vi "get-wakeup-timestamp.vi"(1 "Tga":dbl format="%#_13g", 2 "Tra":dbl format="%#_13g") -> (0 "wake-up timestamp":timestamp)   [LabVIEW 2021]
panel:
  out "current time":timestamp
  # "pre-determined sleep time\nin seconds"
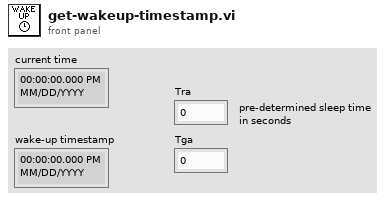
[diagram p1: front panel]
types:
  T1 = typedef "LVDateTimeRec.ctl" = cluster{"fractional second":dbl, "second":i32, "minute":i32, "hour":i32, "day of month":i32, "month":i32, "year":i32, "day of week":i32, "day of year":i32, "DST":i32}
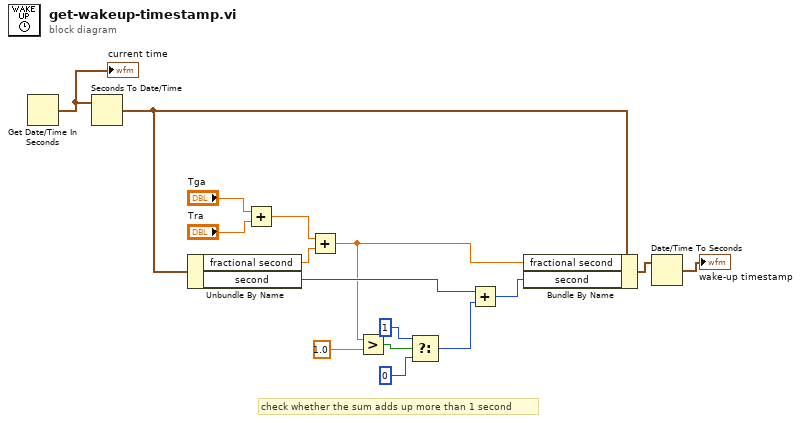
[diagram p0: block diagram]
diagram:
  # "check whether the sum adds up more than 1 second"
  n1 = Get Date/Time In Seconds() -> (seconds since 1Jan1904=w16:timestamp)
  "current time" <- w16
  n2 = Seconds To Date/Time(time stamp (now)=w16) -> (date time rec=w15:T1)  [unwired: 1 in]
  n3 = Unbundle By Name(w15) -> ("fractional second"=w5:dbl, "second"=w6:i32)
  n4 = Add(x="Tga", y="Tra") -> (x+y=w1:dbl)
  n5 = Add(x=w1, y=w5) -> (x+y=w4:dbl)
  n6 = Greater?(x=w4, y=1.0) -> (0:w11:bool)
  n7 = Select(t=1 ("second"), s=w11, f=0 ("second")) -> (s? t:f=w7:i32)
  n8 = Add(x=w6, y=w7) -> (x+y=w8:i32)
  n9 = Bundle By Name(cluster=w15, "fractional second"=w4, "second"=w8) -> (w14:T1)
  n10 = Date/Time To Seconds(2:w14) -> (0:→"wake-up timestamp":timestamp)  [unwired: 1 in]
